vi "DoneWebsocketMessageBroker.vi"(8 "error in (no error)":errorcluster, 11 "Websocket Message Broker Interface Ref in":refnum<class "Websocket Message Broker Interface Ref.lvclass">) -> (0 "error out":errorcluster, 3 "Websocket Message Broker Interface Ref out":refnum<class "Websocket Message Broker Interface Ref.lvclass">)   [LabVIEW 2016, in "Stream Mediator.lvlib" / "Websocket Message Broker Interface Ref.lvclass"]
doc: "--\nCopyright © 2017 Composed SystemsI All rights reserved.\n\nAuthor: Jon McBee <jon.mcbee@composed.io>\n\nThis library is provided \"AS IS\" ,WITHOUT WARRANTIES OR\nCONDITIONS OF ANY KIND, either express or implied.\n\nComposed Systems -- composed.io\n\nStream 0.0.1.1\nJon McBee - Composed Systems\nCopyright (c) 2017, Composed Systems"
uses:
  <userlib>/Composed Systems/Stream/Mediator/Classes/Websocket Message Broker Interface Ref/Websocket Message Broker Interface Ref.lvclass
  C:/Program Files (x86)/National Instruments/LabVIEW 2016/user.lib/Composed Systems/Stream/Mediator/Classes/Message Broker Interface Ref/Message Broker Interface Ref.lvclass
  <userlib>/Composed Systems/Stream/Mediator/Classes/Websocket Message Broker Interface Ref/Websocket Message Broker Interface Ref.lvclass/Websocket Message Broker Interface Ref.ctl
  <userlib>/Composed Systems/Stream/Mediator/Classes/Message Command Stop/Stop Msg.lvclass
  <userlib>/Composed Systems/Stream/Mediator/Classes/Message Broker Interface Ref/Message Broker Interface Ref.lvclass
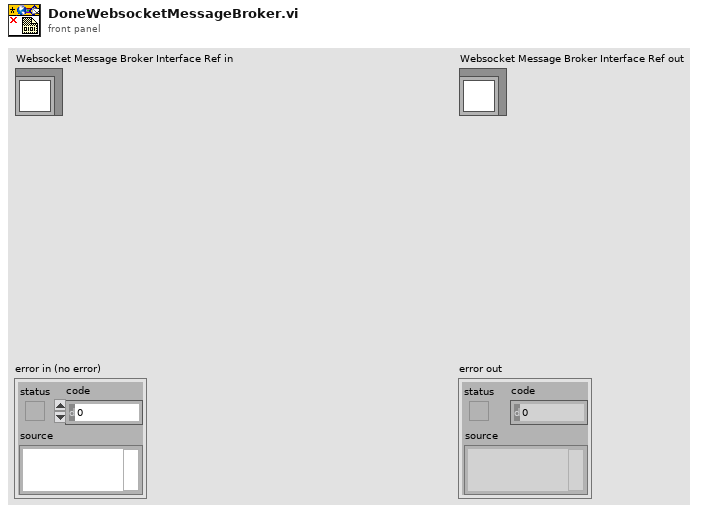
[diagram p1: front panel]
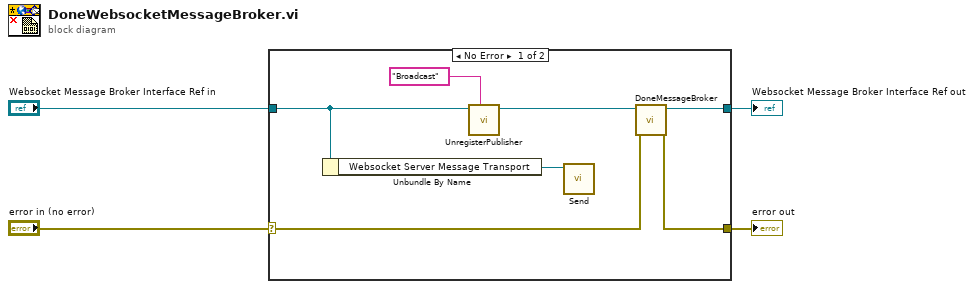
[diagram p0: block diagram]
diagram:
  n1 = case shown="No Error" "error in (no error)" {
    selector: "error in (no error)" -> [w8 w13]
    tunnel: [w7 w13] -> w3
    tunnel: [w9 w12] -> w1
    tunnel: "Websocket Message Broker Interface Ref in" -> [w10 w12]
    frame No Error {
      n2 = Unbundle By Name(w10) -> ("Websocket Server Message Transport"=w11:refnum<class "Message Transport Interface.lvclass">)
      n3 = call-dynamic "UnregisterPublisher.vi"("Topic Name"="Broadcast", "Message Broker Interface TAP in"=w10) -> ("Message Broker Interface TAP out"=w6:refnum<class "Websocket Message Broker Interface Ref.lvclass">)  [unwired: 8 in, 1 out]
      n4 = call <userlib>:"Send.vi"("Message Transport"=w11) -> ()  [unwired: 10 in, 1 out]
      n5 = call <userlib>:"DoneMessageBroker.vi"("error in (no error)"=w8, "Message Broker Interface Ref in"=w6) -> ("error out"=w7:errorcluster, "Message Broker Interface Ref out"=w9:refnum<class "Websocket Message Broker Interface Ref.lvclass">)  [unwired: 8 in]
    }
    frame Error {
    }
  }
  "error out" <- w3
  "Websocket Message Broker Interface Ref out" <- w1
